vi "NI.myDevice main.vi"(6 "Developer Register":refnum<k21>, 7 "NI.myDevice.User Register":refnum<k21>, 8 "NI.myDevice.Serial Interface":cluster{"TX":refnum<k21>, "RX":refnum<k21>}, 9 "NI.myDevice.SPI Interface":T1, 10 "NI.myDevice.Serial Settings":cluster{"slaveID":i16, "baud rate":i16}, 11 "NI.myDevice.Enable Transmission":bool) -> ()   [LabVIEW 2017]
doc: "{Description}\n\n<b>Associated Custom Device</b>\n{Custom Device Name}\n\n<b>Developer</b>\n{Developer Company}\n(Developer Name}\n{Developer Email}"
panel:
  # "All references should be passed in to your VI so they are configurable by the FPGA Developer in the top-level FPGA VI. The resource manager exposes Hardware Resources through the name associated with the project item, but best practices are to give this control the recommended resource name."
  # "Controls that are intended to be exposed to the user SHOULD have your device name prepended so the input created by the FPGA Developer has the correct default name."
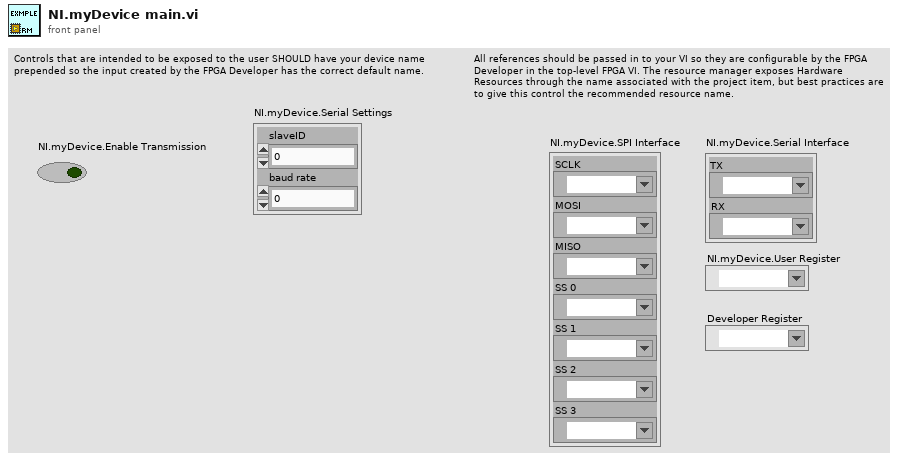
[diagram p1: front panel]
types:
  T1 = cluster{"SCLK":refnum<k21>, "MOSI":refnum<k21>, "MISO":refnum<k21>, "SS 0":refnum<k21>, "SS 1":refnum<k21>, "SS 2":refnum<k21>, "SS 3":refnum<k21>}
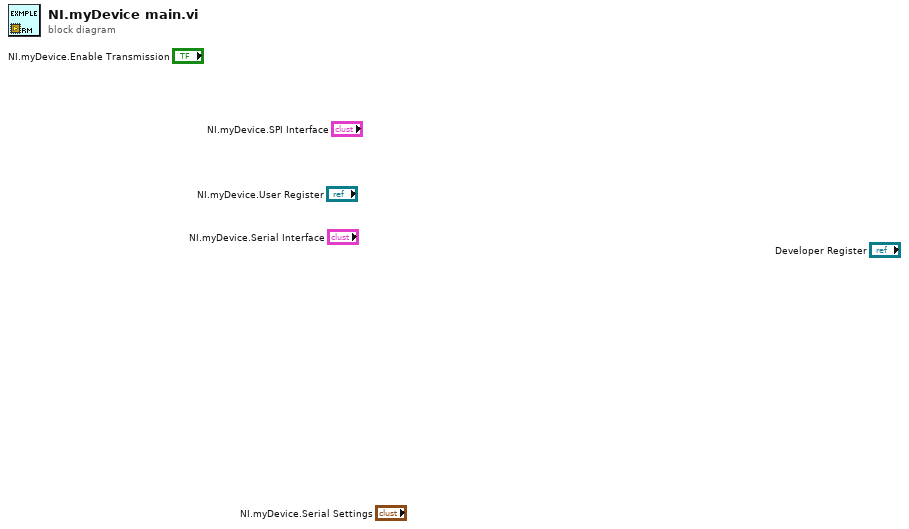
[diagram p0: block diagram]
diagram:
